vi "WRO_Bowling.vi"() -> ()   [LabVIEW 2014]
doc: "The myRIO Project template acquires acceleration data from the onboard accelerometer and displays the changes of acceleration values in a waveform chart."
uses:
  <vilib>/myRIO/Instrument Drivers/Onboard IO/AI/typedefs/AI Reference.ctl
  <vilib>/myRIO/Common/Instrument Driver Framework/Utilities/typedefs/myRIO Generic Hardware Reference.ctl
  <vilib>/myRIO/Common/Instrument Driver Framework/Utilities/typedefs/Hardware Version Enum.ctl
  <vilib>/myRIO/Common/Instrument Driver Framework/Utilities/typedefs/myRIO v1.0 Reference.ctl
  <vilib>/myRIO/Common/Instrument Driver Framework/Utilities/typedefs/Generic FPGA Reference.ctl
  <vilib>/myRIO/Common/Instrument Driver Framework/myRIO v1.0/AI/typedefs/AI Channels List.ctl
  <vilib>/myRIO/Common/Instrument Driver Framework/myRIO v1.0/AI/typedefs/AI Channels Enum.ctl
  <vilib>/myRIO/Common/Instrument Driver Framework/Utilities/typedefs/Analog Scaling Constants List.ctl
  <vilib>/myRIO/Common/Instrument Driver Framework/Utilities/typedefs/Analog Scaling Constants.ctl
  <vilib>/userdefined/High Color/nirio_resource_hc.ctl
  <vilib>/myRIO/Instrument Drivers/Onboard IO/DIO/typedefs/DIO Reference.ctl
  <vilib>/myRIO/Common/Instrument Driver Framework/myRIO v1.0/DIO/typedefs/DIO Channels List.ctl
  <vilib>/myRIO/Common/Instrument Driver Framework/myRIO v1.0/DIO/typedefs/DIO Channels Enum.ctl
  <vilib>/myRIO/Common/Instrument Driver Framework/Utilities/vis/Is FPGA Ref Available.vi
  <vilib>/myRIO/Common/Instrument Driver Framework/myRIO v1.0/AI/vis/myRIO v1.1 Open AI.vi
  <vilib>/myRIO/Instrument Drivers/Onboard IO/AI/vis/Read.vi
  <vilib>/myRIO/Common/Instrument Driver Framework/myRIO v1.0/DIO/vis/myRIO v1.1 Open DIO.vi
  <vilib>/myRIO/Instrument Drivers/Onboard IO/DIO/vis/Write.vi
  <vilib>/myRIO/Common/Instrument Driver Framework/Utilities/vis/Validate Channels.vi
  <vilib>/myRIO/Common/Instrument Driver Framework/myRIO v1.0/AI/vis/myRIO v1.0 Reserve AI.vi
  <vilib>/myRIO/Common/Instrument Driver Framework/myRIO v1.0/DIO/vis/myRIO v1.0 Reserve DIO.vi
  <vilib>/myRIO/Common/Instrument Driver Framework/myRIO v1.0/AI/vis/myRIO v1.0 Build MUX Configuration AI.vi
  <vilib>/myRIO/Common/Instrument Driver Framework/myRIO v1.0/Resource Manager/vis/myRIO v1.0 Reserve Channel List.vi
  <vilib>/myRIO/Common/Instrument Driver Framework/myRIO v1.0/DIO/vis/myRIO v1.0 Build MUX Configuration DIO.vi
  <vilib>/myRIO/Common/Instrument Driver Framework/myRIO v1.0/Resource Manager/vis/myRIO v1.0 Reserve Channel.vi
  <vilib>/myRIO/Common/Instrument Driver Framework/myRIO v1.0/Resource Manager/vis/myRIO v1.0 Unreserve Channel.vi
  <vilib>/myRIO/Common/Instrument Driver Framework/myRIO v1.0/Resource Manager/vis/myRIO v1.0 Create Configuration List.vi
  <vilib>/myRIO/Common/Instrument Driver Framework/myRIO v1.0/Resource Manager/vis/myRIO v1.0 Build Mutex Name.vi
  <vilib>/Utility/VariantDataType/GetNumericInfo.vi
  <vilib>/Utility/error.llb/Error Cluster From Error Code.vi
  <vilib>/myRIO/Common/Instrument Driver Framework/myRIO v1.0/myRIO v1.1 Open.vi
  <vilib>/myRIO/Common/Instrument Driver Framework/myRIO v1.0/AI/vis/myRIO v1.0 Get Scaling Constants AI.vi
  <vilib>/myRIO/Common/Instrument Driver Framework/Utilities/vis/IO Manager.vi
  <vilib>/myRIO/Common/Instrument Driver Framework/Utilities/vis/Configuration Manager.vi
  <vilib>/myRIO/Common/Instrument Driver Framework/myRIO v1.0/myRIO v1.0 Close.vi
  <vilib>/myRIO/Common/Instrument Driver Framework/myRIO v1.0/AI/vis/myRIO v1.0 Read AI.vi
  <vilib>/myRIO/Common/Instrument Driver Framework/myRIO v1.0/Resource Manager/vis/myRIO v1.0 Configure IO.vi
  <vilib>/myRIO/Common/Instrument Driver Framework/myRIO v1.0/DIO/vis/myRIO v1.0 Write DIO.vi
  <vilib>/myRIO/Express VI/Onboard IO/AI/AI Express VI.xnode
  <vilib>/myRIO/Instrument Drivers/Onboard IO/AI/vis/myRIO AI Open.xnode
  <vilib>/myRIO/Express VI/Onboard Devices/LED/LED Express VI.xnode
  <vilib>/myRIO/Instrument Drivers/Onboard IO/DIO/vis/myRIO DIO Open.xnode
  <vilib>/vision/driver/NI_Vision_Acquisition_Software.lvlib
  <vilib>/vision/NI_Vision_Development_Module.lvlib
  <vilib>/myRIO/Instrument Drivers/Onboard IO/AI/AI.lvlib
  <vilib>/myRIO/Instrument Drivers/Onboard IO/DIO/DIO.lvlib
panel:
  out "볼링핀을찾았는가":bool
  in  "Manual":cluster{sgl, sgl}(slide)={0.0, 89.25} caption="Threshold Range" scale=0.0..255.0
  in  "화면전환":bool
  out "Image 3":T1(plugin-control)
  in  "Number of Erosion 2":i32=10
  in  "숫자형 2":dbl=10.0
  in  "y 2":dbl=60.0
  in  "숫자형":dbl
  in  "탭 컨트롤":enum32{"볼링핀 0", "배경 1", "녹색핀 2"}(tab)
  in  "Blue or Luminance":cluster{i32, i32}(slide)={190, 255} scale=0.0..255.0
  in  "Green or Saturation":cluster{i32, i32}(slide)={0, 70} scale=0.0..255.0
  in  "Red or Hue":cluster{i32, i32}(slide)={0, 255} scale=0.0..255.0
  in  "Blue or Luminance 2":cluster{i32, i32}(slide)={0, 145} scale=0.0..255.0
  in  "Green or Saturation 2":cluster{i32, i32}(slide)={1, 41} scale=0.0..255.0
  in  "Red or Hue 2":cluster{i32, i32}(slide)={0, 255} scale=0.0..255.0
  in  "Blue or Luminance 3":cluster{i32, i32}(slide)={60, 255} scale=0.0..255.0
  in  "Green or Saturation 3":cluster{i32, i32}(slide)={35, 255} scale=0.0..255.0
  in  "Red or Hue 3":cluster{i32, i32}(slide)={50, 130} scale=0.0..255.0
  out "초음파센서":bool
  out "Acceleration 4":dbl(graph)=2.6904299629999997
  out "초음파":dbl=2002.725201489796
  out "Acceleration 3":dbl(graph)=2002.725201489796
  in  "y":i16=20
  in  "Number of Erosion":i32=2
  in  "Threshold Color Mode":enum32{"RGB", "HSL"}(radio)=enum."HSL"
  out "Image 2":T1(plugin-control)
  in  "Stop 2":bool
  out "Image":T1(plugin-control)
  in  "Camera Name":refnum<k21>="cam3" caption="IMAQdx Session"
  # "Control Motor"
  # "Read Encoder"
  # "흰색 : 0/255"
  # "흰색 : 0/70~140"
  # "흰색 : 160~190/255"
  # "흰색 : 0/255"
  # "흰색 : 0/90"
  # "흰색 : 170/255"
  # "녹색 : 50/130"
  # "녹색 : 35/255"
  # "녹색 : 60/255"
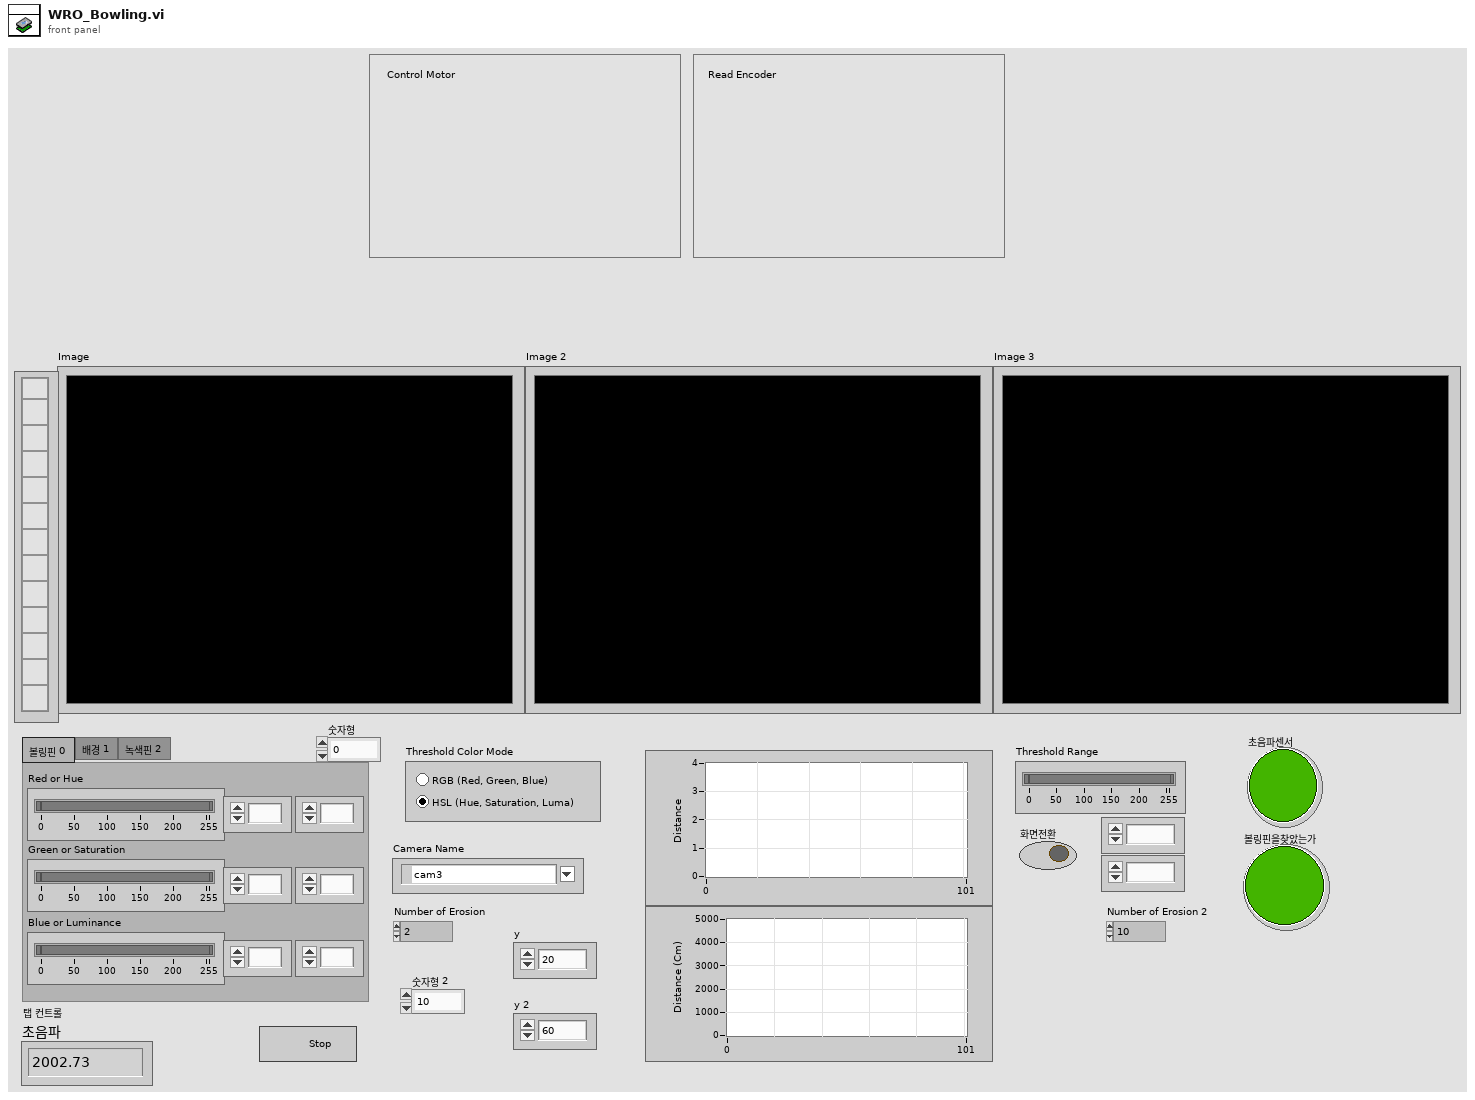
[diagram p1: front panel]
types:
  T1 = typedef "IMAQ Image.ctl" = refnum<image>
  T2 = typedef "DIO.lvlib/DIO Reference.ctl" = cluster{"myRIO Reference":T3, "DIO Channels List":T7}
  T3 = typedef "myRIO Generic Hardware Reference.ctl" = cluster{"myRIO Model":T4, "myRIO Hardware Reference":T5}
  T4 = typedef "Hardware Version Enum.ctl" = enum16{"Unknown", "myRIO-1900", "myRIO-1950"}
  T5 = typedef "myRIO v1.0 Reference.ctl" = cluster{"Generic FPGA Reference":T6, "Allow multiple opens":bool}
  T6 = typedef "Generic FPGA Reference.ctl" = refnum<k20>
  T7 = typedef "DIO Channels List.ctl" = T8[]
  T8 = typedef "DIO Channels Enum.ctl" = enum16{"Not Connected", "C/DIO0", "C/DIO1", "C/DIO2", "C/DIO3", "C/DIO4", "C/DIO5", "C/DIO6", "C/DIO7", "A/DIO0", "A/DIO1", "A/DIO2", "A/DIO3", "A/DIO4", "A/DIO5", "A/DIO6", "A/DIO7", "A/DIO8", "A/DIO9", "A/DIO10", "A/DIO11", "A/DIO12", "A/DIO13", "A/DIO14", "A/DIO15", "B/DIO0", "B/DIO1", "B/DIO2", "B/DIO3", "B/DIO4", "B/DIO5", "B/DIO6", "B/DIO7", "B/DIO8", "B/DIO9", "B/DIO10", "B/DIO11", "B/DIO12", "B/DIO13", "B/DIO14", "B/DIO15", "LED0", "LED1", "LED2", "LED3", "Button0"}
  T9 = typedef "nirio_resource_hc.ctl" = tag
  T10 = typedef "AI.lvlib/AI Reference.ctl" = cluster{"myRIO Reference":T3, "AI Channels List":T11, "AI Scaling Constants List":T13}
  T11 = typedef "AI Channels List.ctl" = T12[]
  T12 = typedef "AI Channels Enum.ctl" = enum16{"Not Connected", "AudioIn/Left", "AudioIn/Right", "C/AI0", "C/AI1", "A/AI0", "A/AI1", "A/AI2", "A/AI3", "B/AI0", "B/AI1", "B/AI2", "B/AI3"}
  T13 = typedef "Analog Scaling Constants List.ctl" = T14[]
  T14 = typedef "Analog Scaling Constants.ctl" = cluster{"LSB Weight (Volts)":dbl, "Offset (Volts)":dbl, "Signed?":bool}
  T15 = typedef "IMAQ Rectangle" = cluster{"Left":i32, "Top":i32, "Right":i32, "Bottom":i32, "Rotation":dbl}
  T16 = typedef "Image Type" = u32
  T17 = typedef "IMAQdx.ctl" = refnum<k21>
  T18 = cluster{"Global Rectangle":i32[], "Contours":cluster{"Contour Type":u32, "ROI Type":u32, "Points":i32[]}[]}
  T19 = cluster{"Area":dbl, "Number of Holes":dbl, "Bounding Rect":cluster{"Left":dbl, "Top":dbl, "Right":dbl, "Bottom":dbl}, "Center of Mass":cluster{"X":dbl, "Y":dbl}, "Orientation":dbl, "Dimensions":cluster{"Width":dbl, "Height":dbl}}[]
  T20 = cluster{"Area":dbl, "Number of Holes":dbl, "Bounding Rect":cluster{"Left":dbl, "Top":dbl, "Right":dbl, "Bottom":dbl}, "Center of Mass":cluster{"X":dbl, "Y":dbl}, "Orientation":dbl, "Dimensions":cluster{"Width":dbl, "Height":dbl}}
  T21 = cluster{"Left":dbl, "Top":dbl, "Right":dbl, "Bottom":dbl}
  T22 = typedef "ROI Descriptor" = cluster{"Global Rectangle":i32[], "Contours":cluster{"ID":enum32{"External", "Internal"}, "Type":u32, "Coordinates":i32[]}[]}
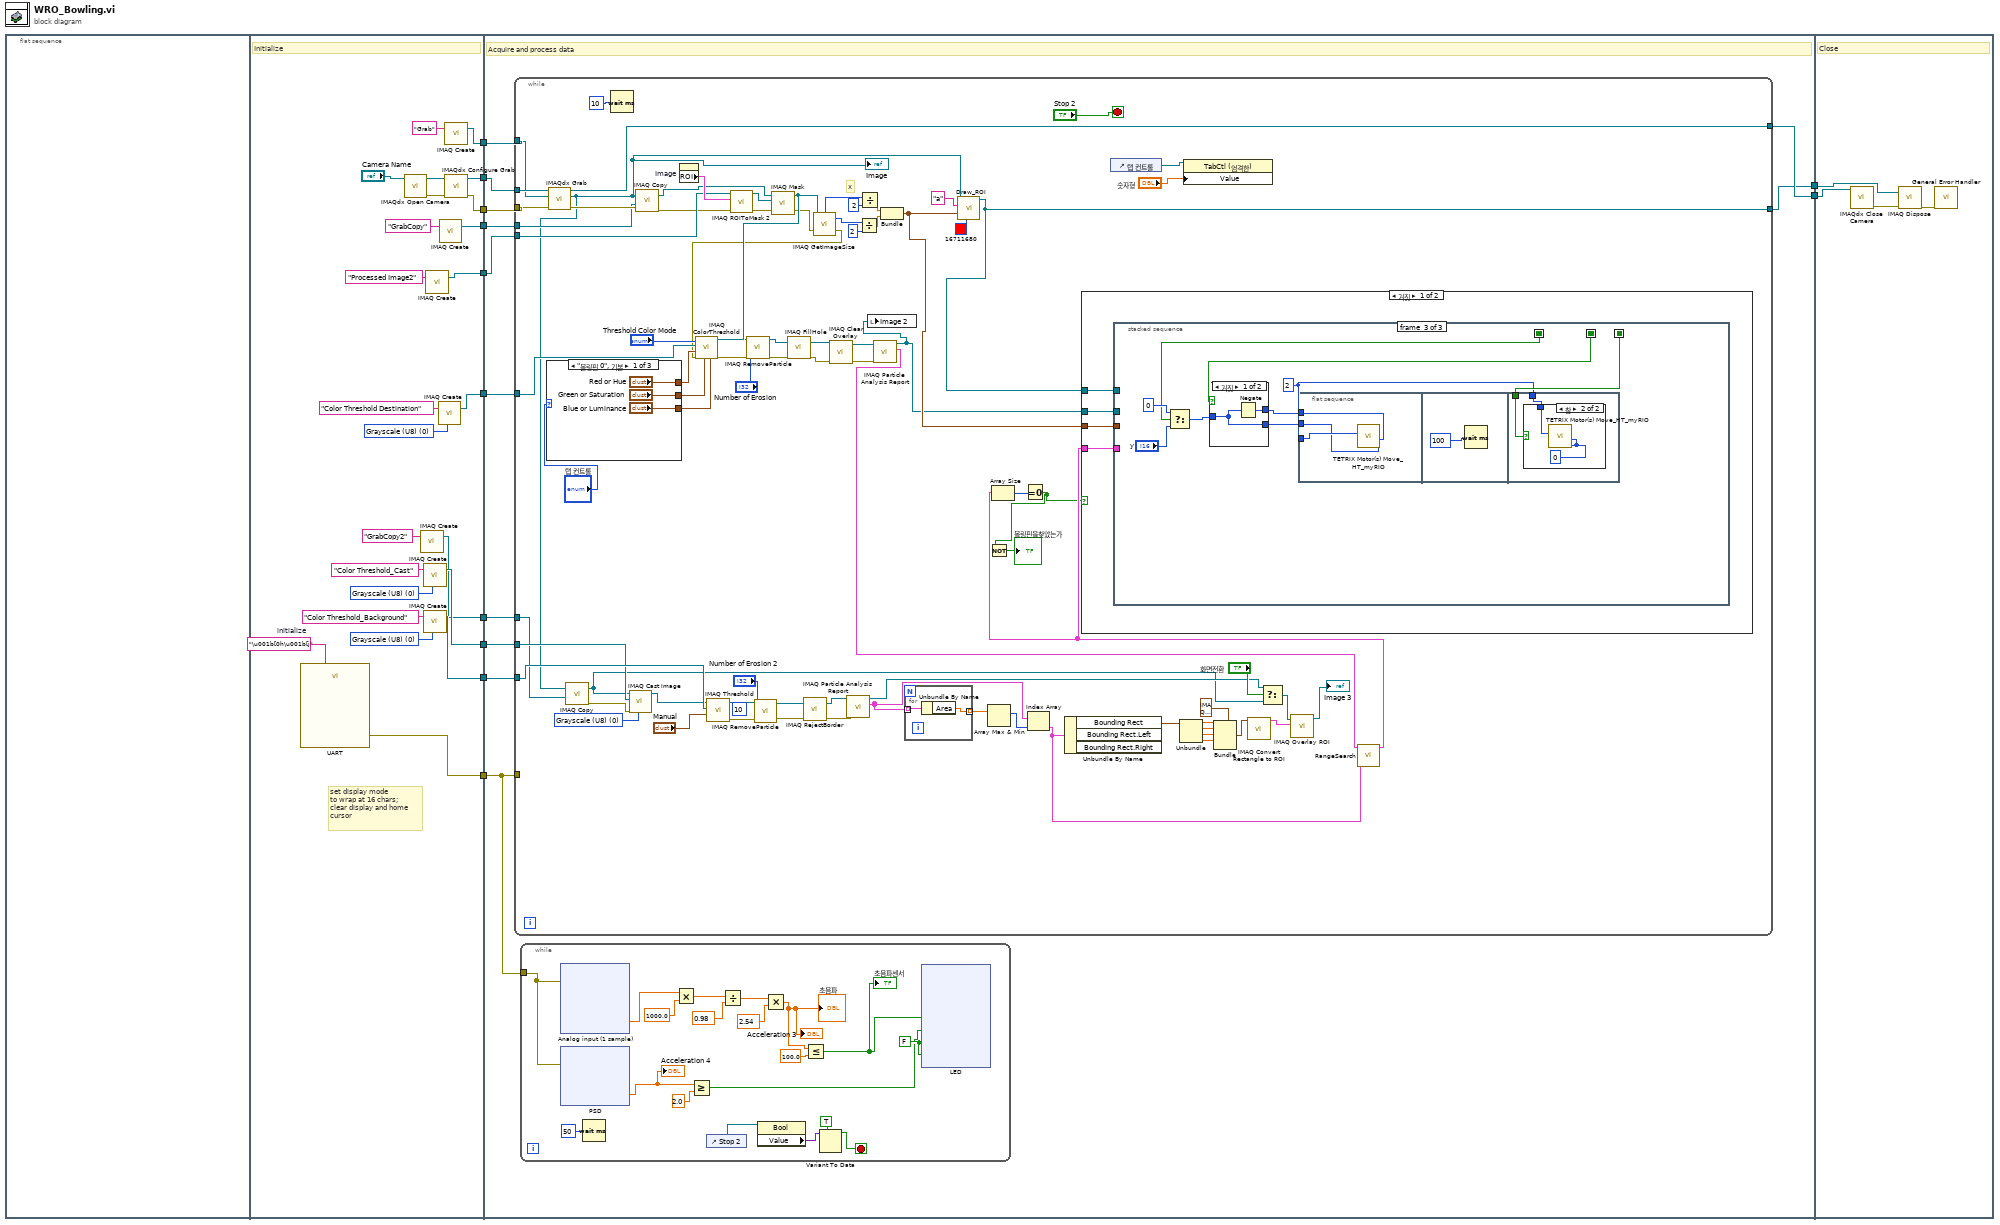
[diagram p0: block diagram]
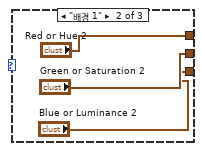
[diagram p2: hidden frame]
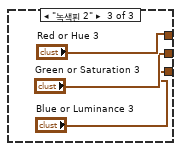
[diagram p3: hidden frame]
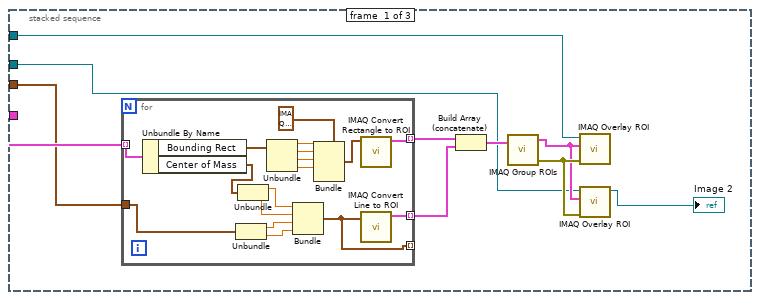
[diagram p4: hidden frame]
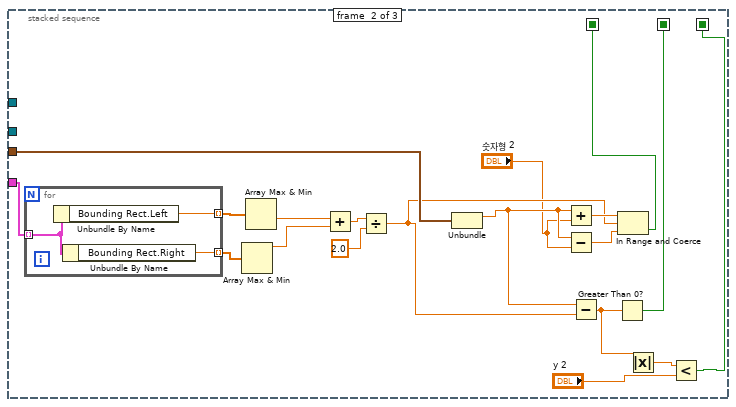
[diagram p5: hidden frame]
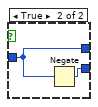
[diagram p7: hidden frame]
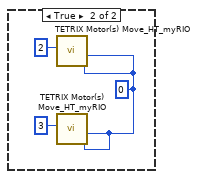
[diagram p8: hidden frame]
diagram:
  n1 = flat-sequence {
    tunnel: [w32] -> w12
    tunnel: [w31] -> w11
    tunnel: [w30] -> w10
    tunnel: [w28] -> w7
    tunnel: [w26] -> w6
    tunnel: [w25] -> w5
    tunnel: [w22] -> w4
    tunnel: [w18] -> w3
    tunnel: [w15] -> w2
    tunnel: [w13] -> w1
    tunnel: w12 -> [w48]
    tunnel: w11 -> [w47]
    tunnel: w10 -> [w46]
    tunnel: [w42] -> w9
    tunnel: [w45] -> w8
    tunnel: w7 -> [w44]
    tunnel: w6 -> [w43]
    tunnel: w5 -> [w40]
    tunnel: w4 -> [w41]
    tunnel: w3 -> [w39]
    tunnel: w2 -> [w38]
    tunnel: w1 -> [w37]
    tunnel: w9 -> [w351]
    tunnel: w8 -> [w350]
    frame #0 {
    }
    frame #1 {
      w16 = T16 0 items=["Grayscale (U8)", "Grayscale (I16)", "Grayscale (SGL)", "Complex (CSG)", "RGB (U32)", "HSL (U32)", "RGB (U64)", "Grayscale (U16)"] ("Image Type")
      w19 = T16 0 items=["Grayscale (U8)", "Grayscale (I16)", "Grayscale (SGL)", "Complex (CSG)", "RGB (U32)", "HSL (U32)", "RGB (U64)", "Grayscale (U16)"] ("Image Type")
      w21 = "\u001b[0h\u001b[j"  # initialize
      w24 = T16 0 items=["Grayscale (U8)", "Grayscale (I16)", "Grayscale (SGL)", "Complex (CSG)", "RGB (U32)", "HSL (U32)", "RGB (U64)", "Grayscale (U16)"] ("Image Type")
      # "set display mode\nto wrap at 16 chars;\nclear display and home\ncursor"
      # "Initialize"
      n2 = call "UART"("Characters to Write"=w21) -> ("error out"=w25:errorcluster)  [unwired: 25 in, 1 out]
      n3 = call <vilib>:"IMAQdx Open Camera.vi"("Session In"="Camera Name") -> ("error out"=w36:errorcluster, "Session Out"=w35:T17)  [unwired: 2 in, 7 out]
      n4 = call "IMAQ Create"("Image Name"="GrabCopy2") -> ("New Image"=w13:T1)  [unwired: 3 in, 2 out]
      n5 = call "IMAQ Create"("Image Name"="Color Threshold_Cast", "Image Type"=w16) -> ("New Image"=w15:T1)  [unwired: 3 in, 1 out]
      n6 = call "IMAQ Create"("Image Name"="Color Threshold_Background", "Image Type"=w19) -> ("New Image"=w18:T1)  [unwired: 3 in, 1 out]
      n7 = call "IMAQ Create"("Image Name"="Processed Image2") -> ("New Image"=w28:T1)  [unwired: 3 in, 2 out]
      n8 = call "IMAQ Create"("Image Name"="Color Threshold Destination", "Image Type"=w24) -> ("New Image"=w22:T1)  [unwired: 3 in, 1 out]
      n9 = call "IMAQ Create"("Image Name"="GrabCopy") -> ("New Image"=w26:T1)  [unwired: 3 in, 2 out]
      n10 = call "IMAQ Create"("Image Name"="Grab") -> ("New Image"=w32:T1)  [unwired: 3 in, 2 out]
      n11 = call <vilib>:"IMAQdx Configure Grab.vi"("error in"=w36, "Session In"=w35) -> ("error out"=w30:errorcluster, "Session Out"=w31:T17)  [unwired: 8 out]
    }
    frame #2 {
      # "Acquire and process data"
      n12 = while {
        tunnel: [w258] -> w45
        tunnel: w46 -> [w260]
        tunnel: w47 -> [w261]
        tunnel: w48 -> [w259]
        tunnel: w44 -> [w254]
        tunnel: w43 -> [w240]
        tunnel: [w218] -> w42
        tunnel: w40 -> [_]
        tunnel: w41 -> [w237]
        tunnel: w39 -> [w216]
        tunnel: w38 -> [w212]
        tunnel: w37 -> [w191]
        stop <- "Stop 2" stop-if-true
        (unwired) 10 ("Number of Erosion")
        w213 = T16 0 items=["Grayscale (U8)", "Grayscale (I16)", "Grayscale (SGL)", "Complex (CSG)", "RGB (U32)", "HSL (U32)", "RGB (U64)", "Grayscale (U16)"] ("Image Type")
        # "x"
        n13 = case shown="\"볼링핀 0\", 기본" "탭 컨트롤" {
          tunnel: ["Blue or Luminance" "Blue or Luminance 2" "Blue or Luminance 3"] -> w235
          tunnel: ["Red or Hue" "Red or Hue 2" "Red or Hue 3"] -> w234
          tunnel: ["Green or Saturation" "Green or Saturation 2" "Green or Saturation 3"] -> w233
          frame "볼링핀 0", Default {
          }
          frame "배경 1" {
          }
          frame "녹색핀 2" {
          }
        }
        n14 = call <vilib>:"IMAQdx Grab.vi"("error in"=w260, "Image In"=w259, "Session In"=w261) -> ("error out"=w242:errorcluster, "Image Out"=w192:T1, "Session Out"=w258:T17)  [unwired: 1 in, 5 out]
        "Image" <- w192
        n15 = call "IMAQ Copy"("Image Dst"=w191, "Image Src"=w192) -> ("error out"=w190:errorcluster, "Image Dst Out"=w184:T1)  [unwired: 4 in]
        n16 = Wait (ms)(milliseconds to wait=u32 10 ("대기 시간(ms)")) -> ()  [unwired: 1 out]
        n17 = call "IMAQ Cast Image"("Image Type"=w213, "error in (no error)"=w190, "Image Dst"=w212, "Image Src"=w184) -> ("Image Dst Out"=w214:T1)  [unwired: 6 in, 1 out]
        n18 = call "IMAQ Copy"("error in (no error)"=w242, "Image Dst"=w240, "Image Src"=w192) -> ("error out"=w241:errorcluster, "Image Dst Out"=w215:T1)  [unwired: 3 in]
        n19 = property on="Image" class="ImageControl"() -> ("ROI"=w256:T18)  [unwired: 2 in, 2 out]
        n20 = call "IMAQ Threshold"("Range"="Manual", "Image Dst"=w216, "Image Src"=w214) -> ("error out"=w211:errorcluster, "Image Dst Out"=w210:T1)  [unwired: 7 in]
        n21 = call "IMAQ ROIToMask 2"("error in (no error)"=w241, "ROI Descriptor"=w256, "Image"=w254) -> ("error out"=w252:errorcluster, "Image Out"=w253:T1)  [unwired: 6 in, 1 out]
        n22 = call "IMAQ RemoveParticle"("error in (no error)"=w211, "Number of Erosion"="Number of Erosion 2", "Image Src"=w210) -> ("error out"=w206:errorcluster, "Image Dst Out"=w207:T1)  [unwired: 7 in]
        n23 = call "IMAQ Mask"("error in (no error)"=w252, "Image Mask"=w253, "Image Src"=w215) -> ("error out"=w238:errorcluster, "Image Dst Out"=w239:T1)  [unwired: 2 in]
        n24 = call "IMAQ RejectBorder"("error in (no error)"=w206, "Image Src"=w207) -> ("error out"=w205:errorcluster, "Image Dst Out"=w204:T1)  [unwired: 4 in]
        n25 = call "IMAQ GetImageSize"("Image"=w239, "error in (no error)"=w238) -> ("Y Resolution"=w247:i32, "X Resolution"=w250:i32, "error out"=w229:errorcluster)  [unwired: 2 in]
        n26 = call "IMAQ ColorThreshold"("Blue or Luma or Val or Inten Range"=w235, "Green or Sat Range"=w233, "Color Mode"="Threshold Color Mode", "error in (no error)"=w229, "Red or Hue Range"=w234, "Image Dst"=w237, "Image Src"=w239) -> ("error out"=w230:errorcluster, "Image Dst Out"=w232:T1)  [unwired: 3 in]
        n27 = call "IMAQ RemoveParticle"("error in (no error)"=w230, "Number of Erosion"="Number of Erosion", "Image Src"=w232) -> ("error out"=w225:errorcluster, "Image Dst Out"=w226:T1)  [unwired: 7 in]
        n28 = call "IMAQ FillHole"("error in (no error)"=w225, "Image Src"=w226) -> ("error out"=w228:errorcluster, "Image Dst Out"=w227:T1)  [unwired: 4 in]
        n29 = call "IMAQ Clear Overlay"("error in (no error)"=w228, "Image"=w227) -> ("error out"=w251:errorcluster, "Image Out"=w257:T1)  [unwired: 1 in, 7 out]
        n30 = call "IMAQ Particle Analysis Report"("error in (no error)"=w205, "Image"=w204) -> ("Particle Reports (Pixels)"=w202:T19, "Image Out (duplicate)"=w188:T1)  [unwired: 4 in, 4 out]
        n31 = Divide(x=w247, y=2) -> (x/y=w245:dbl)
        n32 = Divide(x=w250, y=2) -> (x/y=w246:dbl)
        n33 = call "IMAQ Particle Analysis Report"("error in (no error)"=w251, "Image"=w257) -> ("Particle Reports (Pixels)"=w187:T19, "Image Out (duplicate)"=w208:T1)  [unwired: 4 in, 4 out]
        n34 = local write "Image 2"(w208) -> ()
        n35 = Bundle(w246, w245) -> (w220:cluster{dbl, dbl})  [unwired: 1 in]
        n36 = for {
          tunnel: w202 -> [w263] mode=indexing
          tunnel: [w262] -> w203 mode=indexing
          n37 = Unbundle By Name(w263) -> ("Area"=w262:dbl)
        }
        n38 = call "Draw_ROI.vi"("Color"=u32 16711680, "클러스터"=w220, "Group"="a", "참조 번호 입력"=w192) -> ("참조 번호 출력"=w218:T1)  [unwired: 7 in]
        n39 = Array Max & Min(array=w203) -> (max index (indices)=w201:i32)  [unwired: 3 out]
        n40 = Index Array(array=w202, index=w201) -> (element=w186:T20)
        n41 = Unbundle By Name(w186) -> ("Bounding Rect"=w195:T21)  [unwired: 2 out]
        n42 = control-ref of="탭 컨트롤"() -> (w222:refnum<vi>)
        n43 = Unbundle(w195) -> ("Left"=w196:dbl, "Top"=w197:dbl, "Right"=w198:dbl, "Bottom"=w199:dbl)
        n44 = property class="TabCtl (엄격한)"(reference=w222, "Value"="숫자형") -> ()  [unwired: 1 in, 2 out]
        n45 = Bundle(cluster=T15 {"Left"=0, "Top"=0, "Right"=0, "Bottom"=0, "Rotation"=0.0} ("Rectangle"), "Left"=w196, "Top"=w197, "Right"=w198, "Bottom"=w199) -> (w200:T15)  [unwired: 1 in]
        n46 = call "IMAQ Convert Rectangle to ROI"("Rectangle"=w200) -> ("ROI Descriptor"=w193:T22)  [unwired: 8 in, 1 out]
        n47 = Select(t=w188, s="화면전환", f=w184) -> (s? t:f=w183:T1)
        n48 = call "IMAQ Overlay ROI"("ROI Descriptor"=w193, "Image"=w183) -> ("Image Out"=→"Image 3":T1)  [unwired: 4 in, 5 out]
        n49 = call "RangeSearch.vi"("Particle Report"=w186, "Particle Reports (Pixels)"=w187) -> ("배열"=w185:T19)  [unwired: 9 in]
        n50 = Array Size(array=w185) -> (size(s)=w224:i32)
        n51 = Equal To 0?(x=w224) -> (x = 0?=w180:bool)
        n52 = Not(x=w180) -> (.not. x?=→"볼링핀을찾았는가":bool)
        n53 = case shown="거짓" w180 {
          tunnel: w185 -> [w276 _]
          tunnel: w220 -> [w275 _]
          tunnel: w208 -> [w274 _]
          tunnel: w218 -> [w273 _]
          frame False {
            n54 = stacked-sequence {
              seq-local: [_ w312 _] -> [_ _ w327]
              seq-local: [_ w309 _] -> [_ _ w330]
              seq-local: [_ w305 _] -> [_ _ w328]
              tunnel: w276 -> [w281 w314 _]
              tunnel: w275 -> [w278 w313 _]
              tunnel: w274 -> [w280 _ _]
              tunnel: w273 -> [w279 _ _]
              frame #0 {
                n55 = for {
                  tunnel: w281 -> [w303] mode=indexing
                  tunnel: [w295] -> w283 mode=indexing
                  tunnel: w278 -> [w291]
                  tunnel: [w288] -> w285 mode=indexing
                  tunnel: [w287] -> _ mode=indexing
                  n56 = Unbundle By Name(w303) -> ("Bounding Rect"=w301:T21, "Center of Mass"=w294:cluster{"X":dbl, "Y":dbl})
                  n57 = Unbundle(w291) -> (w290:dbl, w289:dbl)
                  n58 = Unbundle(w294) -> ("X"=w293:dbl, "Y"=w292:dbl)
                  n59 = Unbundle(w301) -> ("Left"=w300:dbl, "Top"=w299:dbl, "Right"=w298:dbl, "Bottom"=w297:dbl)
                  n60 = Bundle("X"=w293, "Y"=w292, w290, w289) -> (w287:cluster{"X":dbl, "Y":dbl, dbl, dbl})  [unwired: 1 in]
                  n61 = Bundle(cluster=T15 {"Left"=0, "Top"=0, "Right"=0, "Bottom"=0, "Rotation"=0.0} ("Rectangle"), "Left"=w300, "Top"=w299, "Right"=w298, "Bottom"=w297) -> (w296:T15)  [unwired: 1 in]
                  n62 = call "IMAQ Convert Rectangle to ROI"("Rectangle"=w296) -> ("ROI Descriptor"=w295:T22)  [unwired: 8 in, 1 out]
                  n63 = call "IMAQ Convert Line to ROI"("Line"=w287) -> ("ROI Descriptor"=w288:T22)  [unwired: 8 in, 1 out]
                }
                n64 = Build Array (concatenate)(w283, w285) -> (w284:T22[])
                n65 = call "IMAQ Group ROIs"("ROI Descriptors"=w284) -> ("error out"=w286:errorcluster, "ROI Descriptor out"=w282:T22)  [unwired: 1 in, 2 out]
                n66 = call "IMAQ Overlay ROI"("error in (no error)"=w286, "ROI Descriptor"=w282, "Image"=w279) -> ()  [unwired: 3 in, 6 out]
                n67 = call "IMAQ Overlay ROI"("error in (no error)"=w286, "ROI Descriptor"=w282, "Image"=w280) -> ("Image Out"=→"Image 2":T1)  [unwired: 3 in, 5 out]
              }
              frame #1 {
                n68 = for {
                  tunnel: w314 -> [w325] mode=indexing
                  tunnel: [w324] -> w319 mode=indexing
                  tunnel: [w323] -> w321 mode=indexing
                  n69 = Unbundle By Name(w325) -> ("Bounding Rect.Left"=w324:dbl)
                  n70 = Unbundle By Name(w325) -> ("Bounding Rect.Right"=w323:dbl)
                }
                n71 = Array Max & Min(array=w321) -> (max value=w322:dbl)  [unwired: 3 out]
                n72 = Array Max & Min(array=w319) -> (min value=w320:dbl)  [unwired: 3 out]
                n73 = Add(x=w320, y=w322) -> (x+y=w315:dbl)
                n74 = Divide(x=w315, y=2.0) -> (x/y=w310:dbl)
                n75 = Unbundle(w313) -> (w311:dbl)  [unwired: 1 out]
                n76 = Add(x=w311, y="숫자형 2") -> (x+y=w317:dbl)
                n77 = Subtract(x=w311, y="숫자형 2") -> (x-y=w318:dbl)
                n78 = Subtract(x=w311, y=w310) -> (x-y=w308:dbl)
                n79 = Greater Than 0?(x=w308) -> (x > 0?=w309:bool)
                n80 = In Range and Coerce(upper limit=w317, x=w310, lower limit=w318) -> (In Range?=w312:bool)  [unwired: 1 out]
                n81 = Absolute Value(x=w308) -> (abs(x)=w307:dbl)
                n82 = Less?(x=w307, y="y 2") -> (x < y?=w305:bool)
              }
              frame #2 {
                w326 = u8 2 ("Controller 2")
                n83 = Select(t=i8 0 ("Motor 2 Power (-100 to 100)\n0 = Stop/Brake\n-128 = Stop/Coast"), s=w327, f="y") -> (s? t:f=w331:i16)
                n84 = case shown="거짓" w330 {
                  tunnel: [w344 w346] -> w334
                  tunnel: w331 -> [w343 w346]
                  tunnel: [w343 w345] -> w333
                  frame False {
                    n85 = Negate(x=w343) -> (-x=w344:i16)
                  }
                  frame True {
                    n86 = Negate(x=w346) -> (-x=w345:i16)
                  }
                }
                n87 = flat-sequence {
                  tunnel: w326 -> [w337]
                  tunnel: w334 -> [w336]
                  tunnel: w333 -> [w335]
                  tunnel: w326 -> [w340]
                  tunnel: w328 -> [w339]
                  frame #0 {
                    n88 = call <vilib>:"TETRIX Motor(s) Move_HT_myRIO.vi"("Motor 2 Power (-100 to 100)\n0 = Stop/Brake\n-128 = Stop/Coast"=w335, "Motor 1 Power (-100 to 100)\n0 = Stop/Brake\n-128 = Stop/Coast"=w336, "Controller Daisy Chain Position: 1 - 4"=w337) -> ()  [unwired: 6 in, 1 out]
                  }
                  frame #1 {
                    n89 = Wait (ms)(milliseconds to wait=u32 100 ("대기 시간(ms)")) -> ()  [unwired: 1 out]
                  }
                  frame #2 {
                    n90 = case shown="참" w339 {
                      tunnel: w340 -> [_ w342]
                      frame False {
                      }
                      frame True {
                        w341 = i8 0 ("Motor 2 Power (-100 to 100)\n0 = Stop/Brake\n-128 = Stop/Coast")
                        n91 = call <vilib>:"TETRIX Motor(s) Move_HT_myRIO.vi"("Motor 2 Power (-100 to 100)\n0 = Stop/Brake\n-128 = Stop/Coast"=w341, "Motor 1 Power (-100 to 100)\n0 = Stop/Brake\n-128 = Stop/Coast"=w341, "Controller Daisy Chain Position: 1 - 4"=w342) -> ()  [unwired: 6 in, 1 out]
                      }
                    }
                  }
                }
              }
            }
          }
          frame True {
            w347 = 0
            n92 = call <vilib>:"TETRIX Motor(s) Move_HT_myRIO.vi"("Motor 2 Power (-100 to 100)\n0 = Stop/Brake\n-128 = Stop/Coast"=w347, "Motor 1 Power (-100 to 100)\n0 = Stop/Brake\n-128 = Stop/Coast"=w347, "Controller Daisy Chain Position: 1 - 4"=u8 2) -> ()  [unwired: 6 in, 1 out]
            n93 = call <vilib>:"TETRIX Motor(s) Move_HT_myRIO.vi"("Motor 2 Power (-100 to 100)\n0 = Stop/Brake\n-128 = Stop/Coast"=w347, "Motor 1 Power (-100 to 100)\n0 = Stop/Brake\n-128 = Stop/Coast"=w347, "Controller Daisy Chain Position: 1 - 4"=u8 3) -> ()  [unwired: 6 in, 1 out]
          }
        }
      }
      n94 = while {
        tunnel: w40 -> [w56]
        stop <- w64 stop-if-true
        w53 = FALSE ("LED1")
        n95 = xnode "Analog input (1 sample)"("error in (no error)"=w56) -> ("UltraSonic (A/AI0 (Pin 3))"=w58:dbl)  [unwired: 1 out]
        n96 = xnode "PSD"("error in (no error)"=w56) -> ("C/AI0 (C/AI0 (AI0))"=w50:dbl)  [unwired: 1 out]
        "Acceleration 4" <- w50
        n97 = Wait (ms)(milliseconds to wait=u32 50 ("대기 시간(ms)")) -> ()  [unwired: 1 out]
        n98 = Multiply(x=w58, y=1000.0) -> (x*y=w61:dbl)
        n99 = Greater Or Equal?(x=w50, y=2.0) -> (x >= y?=w49:bool)
        n100 = control-ref of="Stop 2"() -> (w67:refnum<vi>)
        n101 = Divide(x=w61, y=0.98) -> (x/y=w59:dbl)
        n102 = property class="Bool"(reference=w67) -> ("Value"=w66:variant)  [unwired: 1 in, 2 out]
        n103 = Multiply(x=w59, y=2.54) -> (x*y=w55:dbl)
        "초음파" <- w55
        "Acceleration 3" <- w55
        n104 = Less Or Equal?(x=w55, y=100.0) -> (x <= y?=w52:bool)
        "초음파센서" <- w52
        n105 = Variant To Data(type=TRUE, Variant=w66) -> (data=w64:bool)  [unwired: 1 in, 1 out]
        n106 = xnode "LED"("LED0"=w52, "LED1"=w49, "LED2"=w53, "LED3"=w53) -> ()  [unwired: 1 in, 1 out]
      }
    }
    frame #3 {
      # "Close"
      n107 = call <vilib>:"IMAQdx Close Camera.vi"("Session In"=w350) -> ("error out"=w353:errorcluster)  [unwired: 1 in, 9 out]
      n108 = call "IMAQ Dispose"("Image"=w351, "error in (no error)"=w353) -> ("error out"=w352:errorcluster)  [unwired: 4 in]
      n109 = call <vilib>:"General Error Handler.vi"("error in (no error)"=w352) -> ()  [unwired: 2 in, 13 out]
    }
  }
